vi "Realy Output User Interface.vi"() -> ()   [LabVIEW 2023, in "GUI.lvlib" / "Diagnostic.lvlib"]
uses:
  Diagnostic.lvlib
  Control/Relay Output 2520.ctl
  Digital Output/Control/Digital Output.ctl
  HardwareAbstractionLayer_LVOOP/NI Switch/NISwitch_class/NISwitch.lvclass
  HardwareAbstractionLayer_LVOOP/Database/SQL Public VI/Control/DB Options.ctl
  HardwareAbstractionLayer_LVOOP/Main/Class Ref.ctl
  HardwareAbstractionLayer_LVOOP/DMM/DMM.lvclass
  HardwareAbstractionLayer_LVOOP/Function Generator/Function Generator.lvclass
  HardwareAbstractionLayer_LVOOP/Oscilloscope/Oscilloscope.lvclass
  HardwareAbstractionLayer_LVOOP/PowerSupply/PowerSupply.lvclass
  HardwareAbstractionLayer_LVOOP/Teststand/Teststand.lvclass
  HardwareAbstractionLayer_LVOOP/Analog Output/AO/AO.lvclass
  HardwareAbstractionLayer_LVOOP/Analog Input/AI/AI.lvclass
  HardwareAbstractionLayer_LVOOP/Database/Database.lvclass
  HardwareAbstractionLayer_LVOOP/Digital Output/DO_class/DO.lvclass
  HardwareAbstractionLayer_LVOOP/Digital Input/DI_class/DI.lvclass
  HardwareAbstractionLayer_LVOOP/PWM Output/PWM Output_class/PWM Output.lvclass
  HardwareAbstractionLayer_LVOOP/PWM Input/PWM Input_class/PWM Input.lvclass
  HardwareAbstractionLayer_LVOOP/Modbus/Modbus_class/Modbus.lvclass
  HardwareAbstractionLayer_LVOOP/CAN/CAN Lib/CAN_class/CAN.lvclass
  <instrlib>/niSwitch/niSwitch.llb/niSwitch Relay Action.ctl
  <instrlib>/niSwitch/niSwitch.llb/niSwitch Topologies.ctl
  HardwareAbstractionLayer_LVOOP/Main/Main.lvclass
panel:
  in  "Start Acquire":bool
  in  "Stop Acquire":bool
  out "error out":errorcluster
  in  "error in":errorcluster
  in  "Operation":enum32{"2520PXI2Slot17"}(tab)
  in  "PXI-2520":T1
  in  "Stop":bool caption="Blank"
  in  "Apply":bool caption="Blank"
  # "Relay Output"
  # "Device:"
  # "***Note: Relay Output PXI2520 Card Is Access Simultaneously Accecss any 40 Output Only"
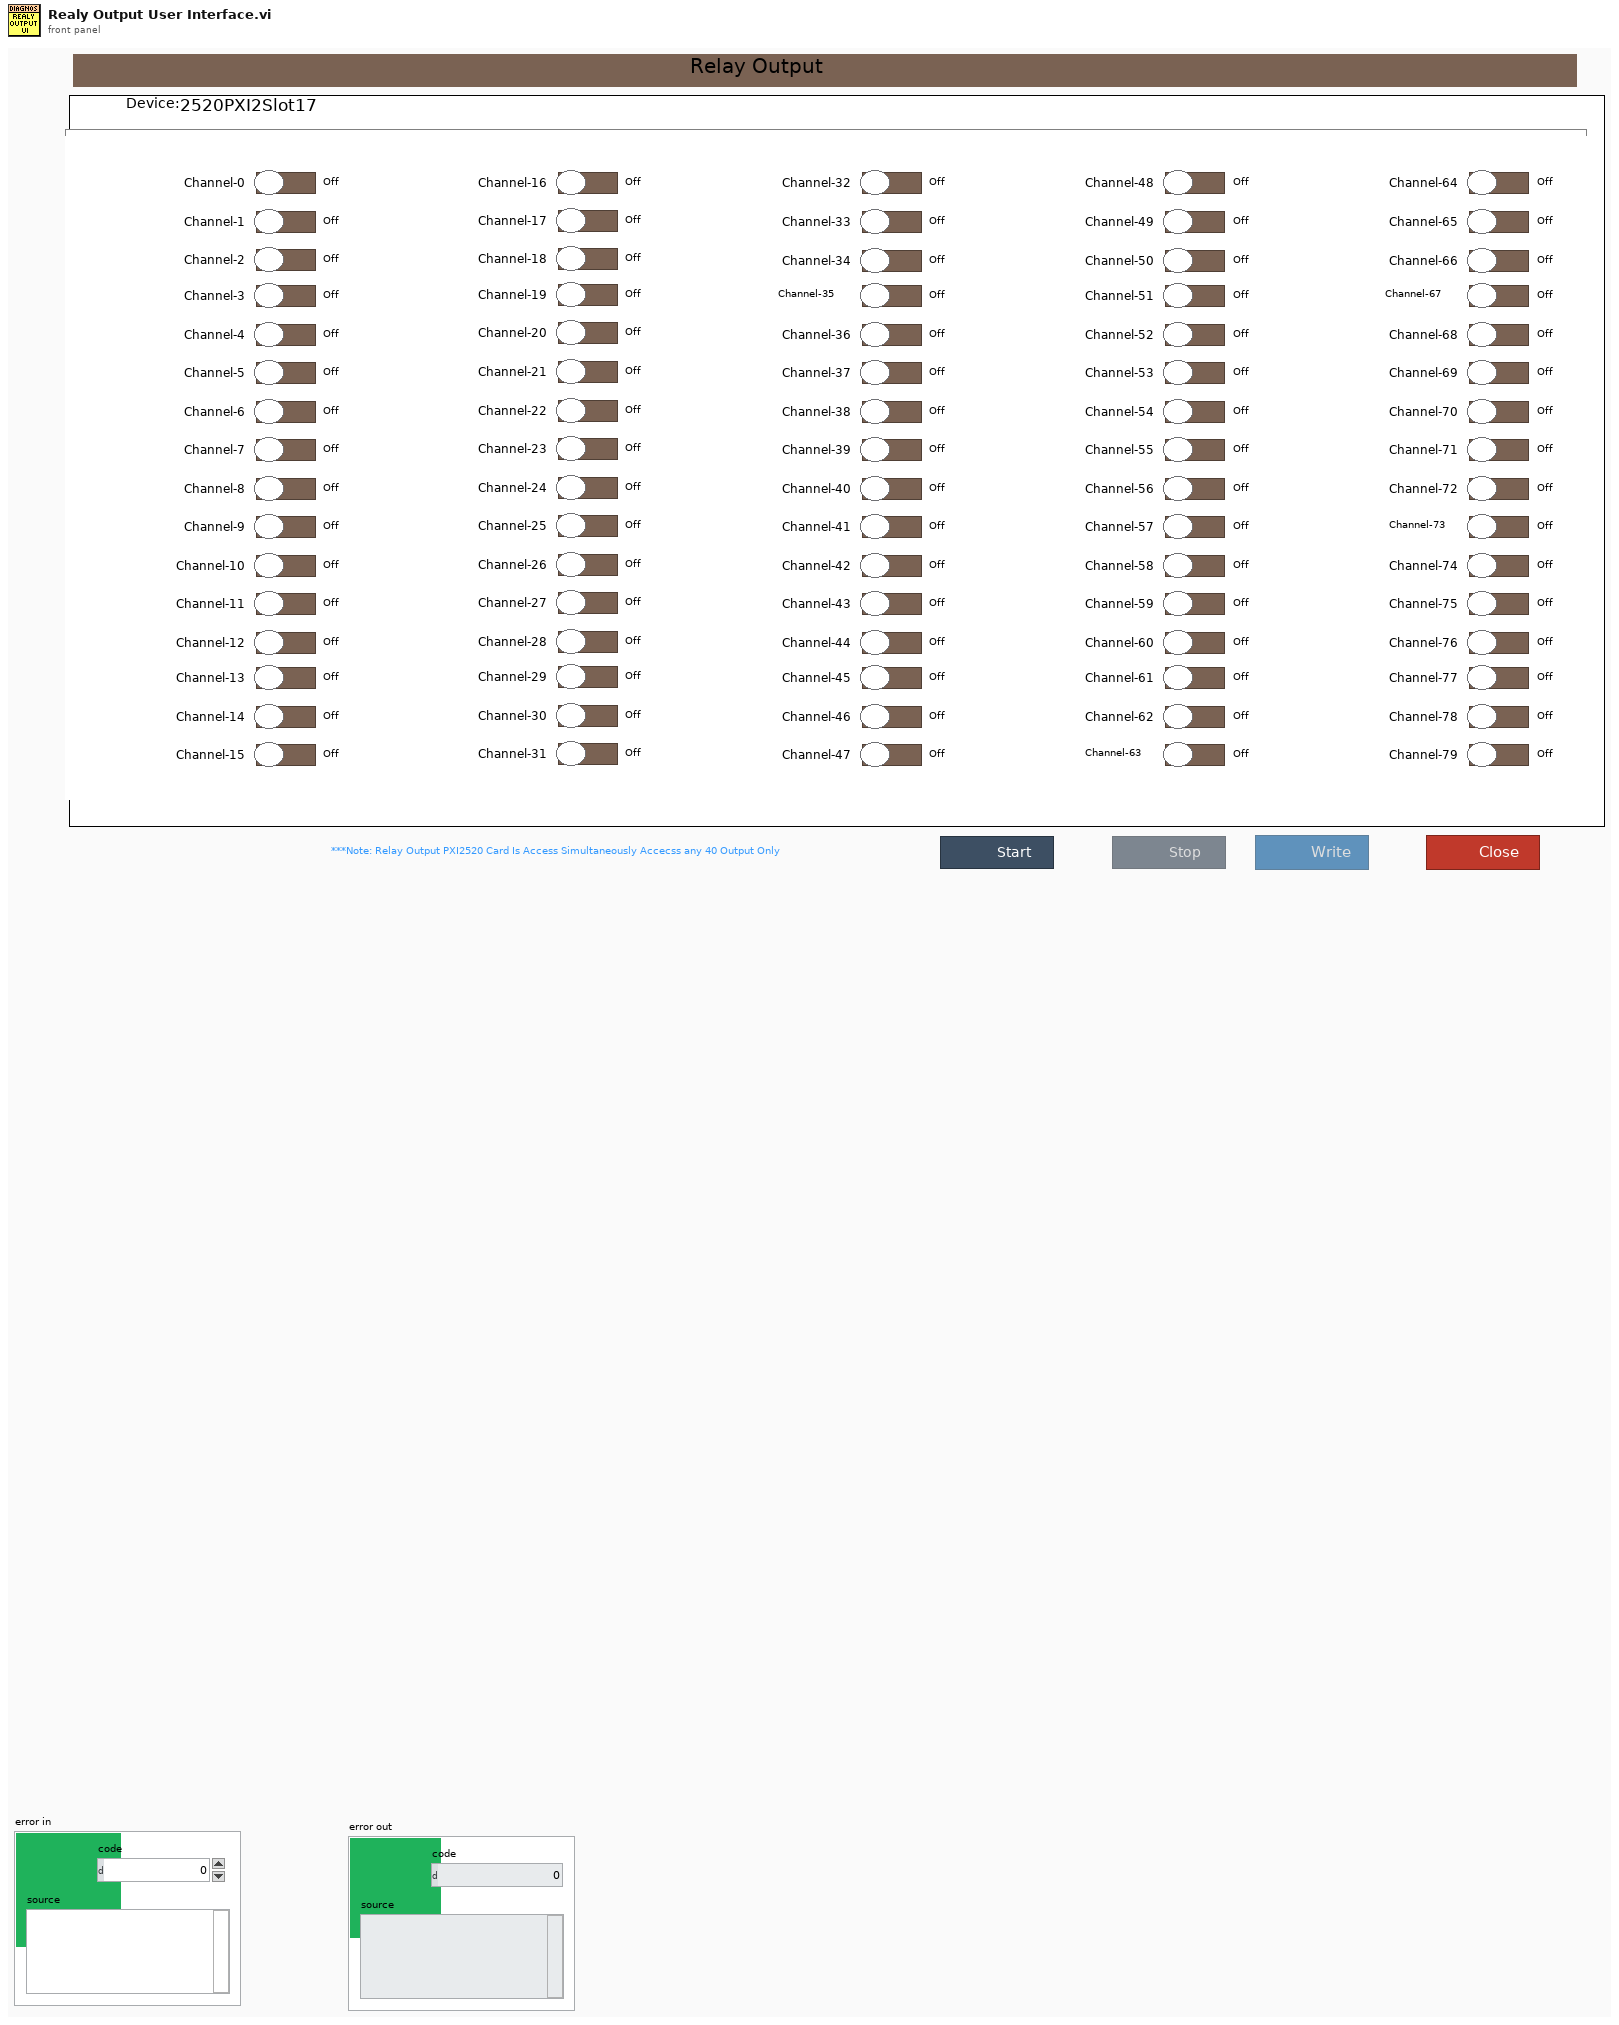
[diagram p1: front panel]
types:
  T1 = typedef "GUI.lvlib/Diagnostic.lvlib/Relay Output 2520.ctl" = cluster{"Channel-0":T2, "Channel-1":T2, "Channel-2":T2, "Channel-3":T2, "Channel-4":T2, "Channel-5":T2, "Channel-6":T2, "Channel-7":T2, "Channel-8":T2, "Channel-9":T2, "Channel-10":T2, "Channel-11":T2, "Channel-12":T2, "Channel-13":T2, "Channel-14":T2, "Channel-15":T2, "Channel-16":T2, "Channel-17":T2, "Channel-18":T2, "Channel-19":T2, "Channel-20":T2, "Channel-21":T2, "Channel-22":T2, "Channel-23":T2, "Channel-24":T2, "Channel-25":T2, "Channel-26":T2, "Channel-27":T2, "Channel-28":T2, "Channel-29":T2, "Channel-30":T2, "Channel-31":T2, "Channel-32":T2, "Channel-33":T2, "Channel-34":T2, "Channel-35":T2, "Channel-36":T2, "Channel-37":T2, "Channel-38":T2, "Channel-39":T2, "Channel-40":T2, "Channel-41":T2, "Channel-42":T2, "Channel-43":T2, "Channel-44":T2, "Channel-45":T2, "Channel-46":T2, "Channel-47":T2, "Channel-48":T2, "Channel-49":T2, "Channel-50":T2, "Channel-51":T2, "Channel-52":T2, "Channel-53":T2, "Channel-54":T2, "Channel-55":T2, "Channel-56":T2, "Channel-57":T2, "Channel-58":T2, "Channel-59":T2, "Channel-60":T2, "Channel-61":T2, "Channel-62":T2, "Channel-63":T2, "Channel-64":T2, "Channel-65":T2, "Channel-66":T2, "Channel-67":T2, "Channel-68":T2, "Channel-69":T2, "Channel-70":T2, "Channel-71":T2, "Channel-72":T2, "Channel-73":T2, "Channel-74":T2, "Channel-75":T2, "Channel-76":T2, "Channel-77":T2, "Channel-78":T2, "Channel-79":T2}
  T2 = typedef "GUI.lvlib/Diagnostic.lvlib/Digital Output.ctl" = bool
  T3 = typedef "HardwareAbstractionLayer_LVOOP.lvlib/Database.lvclass/DB Options.ctl" = enum16{"Init", "Select Data", "Insert Data", "Update Data", "Delete Data", "Execute Query", "Create Schema", "Create Table", "List Tables", "List Columns", "Close"}
  T4 = typedef "HardwareAbstractionLayer_LVOOP.lvlib/Main.lvclass/Class Ref.ctl" = cluster{"DMM":refnum<class "DMM.lvclass">, "Function Generator":refnum<class "Function Generator.lvclass">, "Oscilloscope":refnum<class "Oscilloscope.lvclass">, "PowerSupply":refnum<class "PowerSupply.lvclass">, "Teststand":refnum<class "Teststand.lvclass">, "AO":refnum<class "AO.lvclass">, "AI":refnum<class "AI.lvclass">, "Database":refnum<class "Database.lvclass">, "AO Waveform Generation":refnum<class "AO.lvclass">, "DO":refnum<class "DO.lvclass">, "DI":refnum<class "DI.lvclass">, "PWM Output":refnum<class "PWM Output.lvclass">, "PWM Input":refnum<class "PWM Input.lvclass">, "RelayOutput":refnum<class "NISwitch.lvclass">, "Modbus":refnum<class "Modbus.lvclass">, "CAN":refnum<class "CAN.lvclass">}
  T5 = enum8{"Enabled", "Disabled", "Disabled and Grayed Out"}
  T6 = typedef "niSwitch Topologies.ctl" = string
  T7 = typedef "niSwitch Relay Action.ctl" = i32
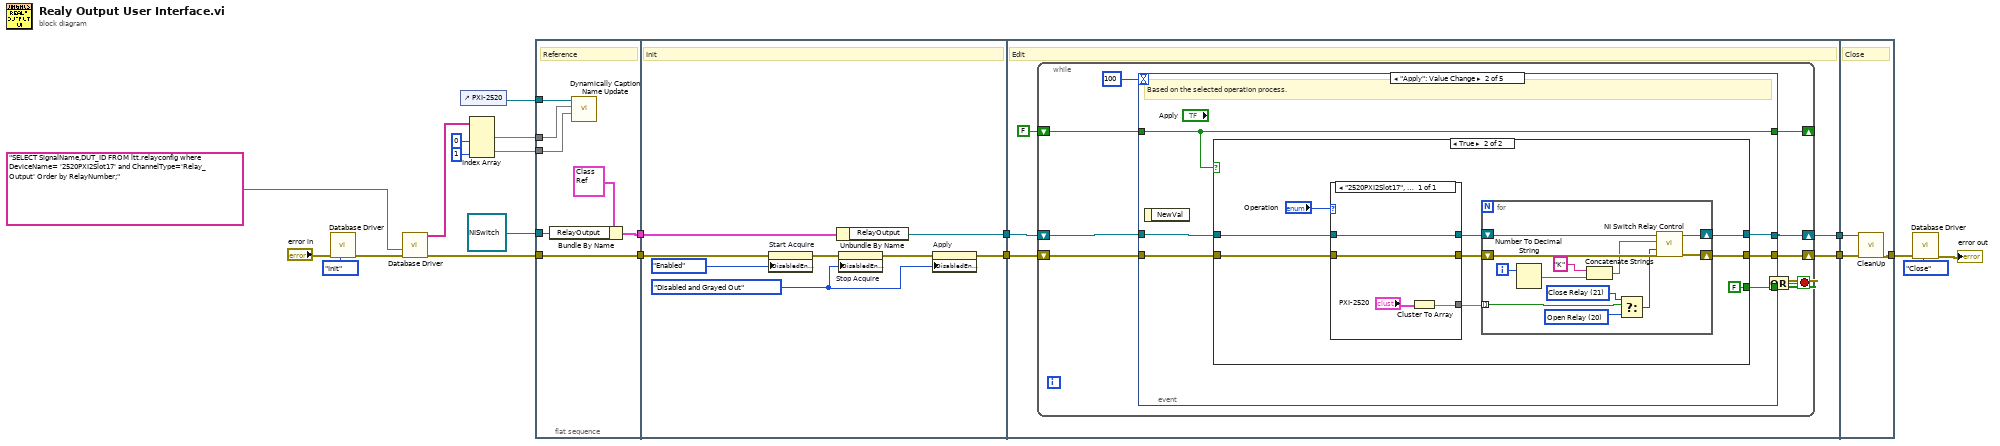
[diagram p0: block diagram]
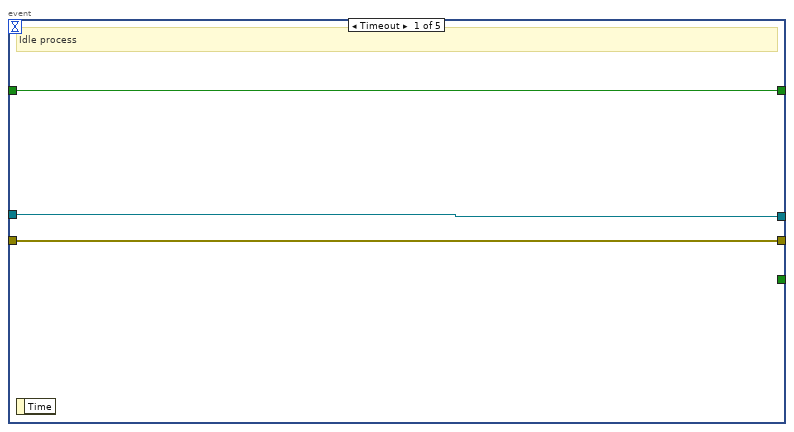
[diagram p2: hidden frame]
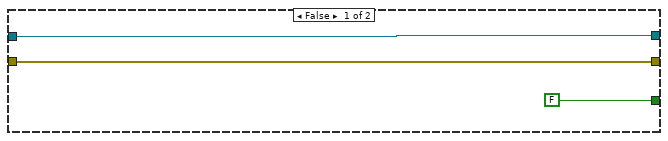
[diagram p3: hidden frame]
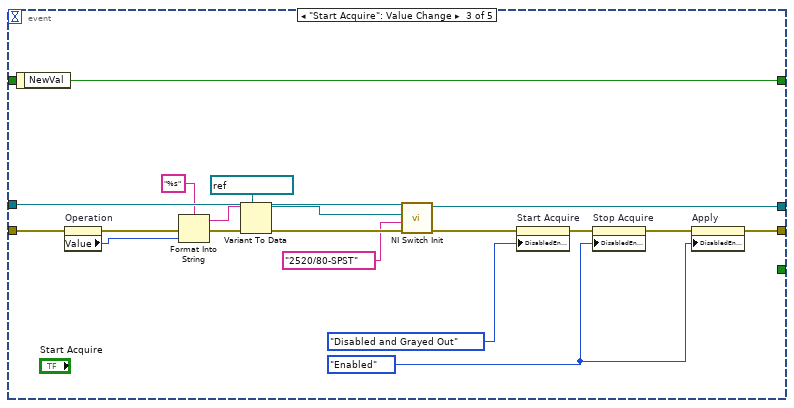
[diagram p4: hidden frame]
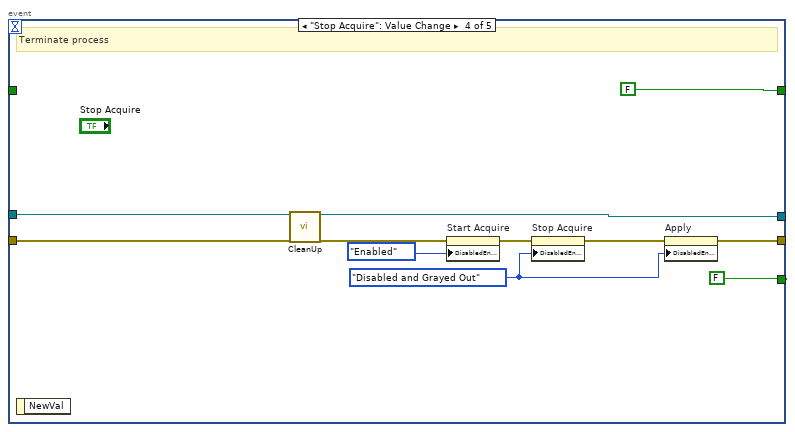
[diagram p5: hidden frame]
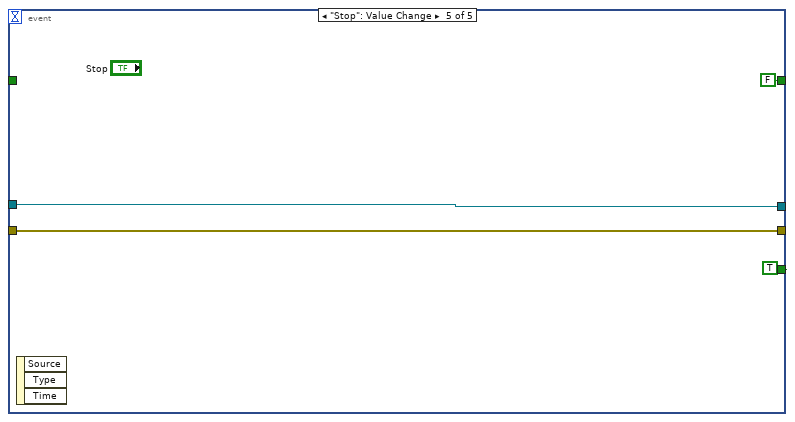
[diagram p6: hidden frame]
diagram:
  n1 = call "Database Driver.vi"("Options"=DB_Options."Init", "error in"="error in") -> ("error out"=w9:errorcluster)  [unwired: 6 in, 3 out]
  n2 = call "Database Driver.vi"("error in"=w9, "SQL query"="SELECT SignalName,DUT_ID FROM ltt.relayconfig where DeviceName= '2520PXI2Slot17' and ChannelType='Relay_Output' Order by RelayNumber;") -> ("error out"=w8:errorcluster, "data"=w6:string[][])  [unwired: 6 in, 2 out]
  n3 = control-ref of="PXI-2520"() -> (w4:refnum<vi>)
  n4 = Index Array(array=w6, index (col) #1=0 ("disabled index (col)"), index (col) #2=1 ("index (col)")) -> (element #1=w3:string[], element #2=w2:string[])  [unwired: 2 in]
  n5 = flat-sequence {
    tunnel: [w27] -> w21
    tunnel: refnum<class "NISwitch.lvclass"> refnum ("HardwareAbstractionLayer_LVOOP.lvlib:RelayOutput") -> [w26]
    tunnel: w8 -> [w25]
    tunnel: [w25] -> w11
    tunnel: w4 -> [w24]
    tunnel: w3 -> [w23]
    tunnel: w2 -> [w22]
    tunnel: w21 -> [w36]
    tunnel: [w35] -> w19
    tunnel: [w30] -> w12
    tunnel: w11 -> [w34]
    tunnel: w19 -> [w40]
    tunnel: [w39] -> w18
    tunnel: [w38] -> w17
    tunnel: w12 -> [w41]
    tunnel: w18 -> [w122]
    tunnel: w17 -> [w124]
    tunnel: [w123] -> w10
    frame #0 {
      # "Reference"
      n6 = Bundle By Name(cluster=T4 {"DMM"=refnum, "Function Generator"=refnum, "Oscilloscope"=refnum, "PowerSupply"=refnum, "Teststand"=refnum, "AO"=refnum, "AI"=refnum, "Database"=refnum, "AO Waveform Generation"=refnum, "DO"=refnum, "DI"=refnum, "PWM Output"=refnum, "PWM Input"=refnum, "RelayOutput"=refnum, "Modbus"=refnum, "CAN"=refnum} ("Class Cluster"), "RelayOutput"=w26) -> (w27:T4)
      n7 = call "Dynamically Caption Name Update.vi"("DUT_Number"=w22, "Caption Name"=w23, "Clust Refnum"=w24) -> ()  [unwired: 8 in, 1 out]
    }
    frame #1 {
      w29 = T5."Disabled and Grayed Out" ("Disabled")
      # "Init"
      n8 = property on="Start Acquire" class="Bool"(error in=w34, "DisabledEnum"=T5."Enabled" ("Disabled")) -> (error out=w33:errorcluster)  [unwired: 1 in, 1 out]
      n9 = Unbundle By Name(w36) -> ("RelayOutput"=w35:refnum<class "NISwitch.lvclass">)
      n10 = property on="Stop Acquire" class="Bool"(error in=w33, "DisabledEnum"=w29) -> (error out=w31:errorcluster)  [unwired: 1 in, 1 out]
      n11 = property on="Apply" class="Bool (strict)"(error in=w31, "DisabledEnum"=w29) -> (error out=w30:errorcluster)  [unwired: 1 in, 1 out]
    }
    frame #2 {
      # "Edit"
      n12 = while {
        shift-right: [w46] -> w38
        shift-left: w40 -> [w47]
        shift-right: [w42] -> w39
        shift-left: w41 -> [w48]
        shift-right: [w45] -> _
        shift-left: FALSE ("NewVal") -> [w44]
        stop <- w43 stop-if-true
        n13 = event shown="[1] \"Apply\": Value Change" {
          selector: _ -> [_ _ _ _ _]
          dyn-events: _ -> [_ _ _ _ _]
          timeout: 100 -> [_ _ _ _ _]
          tunnel: [_ w55 _ FALSE TRUE] -> w50
          tunnel: w48 -> [w52 w58 w90 w115 w120]
          tunnel: w47 -> [w53 w59 w105 w114 w121]
          tunnel: [w52 w57 w99 w108 w120] -> w42
          tunnel: [w53 w56 w104 w113 w121] -> w46
          tunnel: [w51 w54 w106 FALSE ("NewVal") FALSE ("NewVal")] -> w45
          tunnel: w44 -> [w51 w54 _ _ _]
          event Timeout {
            # "Idle process"
            n14 = event-data() -> ()  [unwired: 1 in, 1 out]
          }
          event "Apply": Value Change {
            # "Based on the selected operation process."
            n15 = event-data() -> ()  [unwired: 1 in, 1 out]
            n16 = case shown="True" w54 {
              tunnel: w59 -> [w62 w66]
              tunnel: w58 -> [w61 w65]
              tunnel: [w61 w71] -> w57
              tunnel: [w62 w70] -> w56
              tunnel: [FALSE FALSE] -> w55
              frame False {
              }
              frame True {
                n17 = case shown="\"2520PXI2Slot17\", Default" "Operation" {
                  tunnel: [w74] -> w68
                  tunnel: w66 -> [w72]
                  tunnel: w65 -> [w73]
                  tunnel: [w73] -> w64
                  tunnel: [w72] -> w63
                  frame "2520PXI2Slot17", Default {
                    n18 = Cluster To Array(cluster="PXI-2520") -> (array=w74:T2[])
                  }
                }
                n19 = for {
                  tunnel: w68 -> [w79] mode=indexing
                  shift-right: [w76] -> w70
                  shift-left: w63 -> [w87]
                  shift-right: [w77] -> w71
                  shift-left: w64 -> [w86]
                  i -> [w85]
                  w81 = T7 21 items=["Open Relay"=20, "Close Relay"=21] ("relay action (Close Relay)")
                  w80 = T7 20 items=["Open Relay"=20, "Close Relay"=21] ("relay action (Close Relay)")
                  n20 = Number To Decimal String(number=w85) -> (decimal integer string=w84:string)  [unwired: 1 in]
                  n21 = Concatenate Strings("K" ("string"), w84) -> (w82:string)
                  n22 = Select(t=w81, s=w79, f=w80) -> (s? t:f=w78:T7)
                  n23 = call-dynamic "NI Switch Relay Control.vi"("error in (no error)"=w86, "relay action (Close Relay)"=w78, "relay names"=w82, "RelayOutput in"=w87) -> ("error out"=w77:errorcluster, "RelayOutput out"=w76:refnum<class "NISwitch.lvclass">)  [unwired: 6 in]
                }
              }
            }
          }
          event "Start Acquire": Value Change {
            w98 = T5."Enabled" ("Disabled")
            n24 = event-data() -> ("NewVal"=w106:bool)  [unwired: 1 in]
            n25 = property on="Operation" class="TabCtl (strict)"(error in=w90) -> (error out=w89:errorcluster, "Value"=w88:enum32{"2520PXI2Slot17"})  [unwired: 1 in, 1 out]
            n26 = Format Into String(format string="%s", error in=w89, w88) -> (resulting string=w94:string, error out=w95:errorcluster)  [unwired: 1 in]
            n27 = Variant To Data(error in=w95, type=refnum<k15> "PXI2Slot17" ("resource name"), Variant=w94) -> (data=w92:refnum<k15>, error out=w93:errorcluster)
            n28 = call "NI Switch Init.vi"("error in (no error)"=w93, "topology name"=T6 "2520/80-SPST", "resource name"=w92, "object in"=w105) -> ("error out"=w101:errorcluster, "object out"=w104:refnum<class "NISwitch.lvclass">)  [unwired: 6 in]
            n29 = property on="Start Acquire" class="Bool"(error in=w101, "DisabledEnum"=T5."Disabled and Grayed Out" ("Disabled")) -> (error out=w102:errorcluster)  [unwired: 1 in, 1 out]
            n30 = property on="Stop Acquire" class="Bool"(error in=w102, "DisabledEnum"=w98) -> (error out=w100:errorcluster)  [unwired: 1 in, 1 out]
            n31 = property on="Apply" class="Bool (strict)"(error in=w100, "DisabledEnum"=w98) -> (error out=w99:errorcluster)  [unwired: 1 in, 1 out]
          }
          event "Stop Acquire": Value Change {
            w107 = T5."Disabled and Grayed Out" ("Disabled")
            # "Terminate process"
            n32 = event-data() -> ()  [unwired: 1 in, 1 out]
            n33 = call-dynamic "CleanUp.vi"("object in"=w114, "error in (no error)"=w115) -> ("object out"=w113:refnum<class "NISwitch.lvclass">, "error out"=w110:errorcluster)  [unwired: 16 in]
            n34 = property on="Start Acquire" class="Bool"(error in=w110, "DisabledEnum"=T5."Enabled" ("Disabled")) -> (error out=w111:errorcluster)  [unwired: 1 in, 1 out]
            n35 = property on="Stop Acquire" class="Bool"(error in=w111, "DisabledEnum"=w107) -> (error out=w109:errorcluster)  [unwired: 1 in, 1 out]
            n36 = property on="Apply" class="Bool (strict)"(error in=w109, "DisabledEnum"=w107) -> (error out=w108:errorcluster)  [unwired: 1 in, 1 out]
          }
          event "Stop": Value Change {
            n37 = event-data() -> ()  [unwired: 1 in, 3 out]
          }
        }
        n38 = Compound Arithmetic op=OR(w42, w50) -> (w43:bool)
      }
    }
    frame #3 {
      # "Close"
      n39 = call-dynamic "CleanUp.vi"("object in"=w124, "error in (no error)"=w122) -> ("error out"=w123:errorcluster)  [unwired: 16 in, 1 out]
    }
  }
  n40 = call "Database Driver.vi"("Options"=DB_Options."Close", "error in"=w10) -> ("error out"=→"error out":errorcluster)  [unwired: 6 in, 3 out]
